vi "test_pathClassScalar.vi"(8 "error in (no error)":errorcluster) -> (0 "error out":errorcluster)   [LabVIEW 2020]
uses:
  test-TestableClass/Caraya-TestableClass.lvclass
  run-tests/Run Test (Scalar Path).vi
  Caraya.lvlib
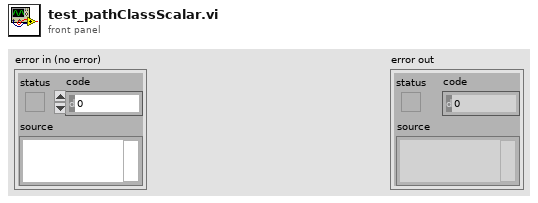
[diagram p1: front panel]
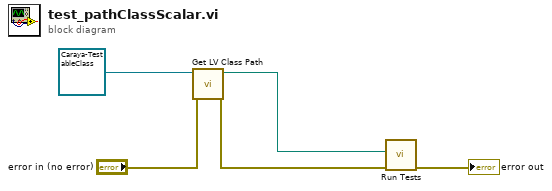
[diagram p0: block diagram]
diagram:
  n1 = call <vilib>:"Get LV Class Path.vi"("error in (no error)"="error in (no error)", "object"=refnum<class "Caraya-TestableClass.lvclass"> refnum ("Caraya-TestableClass.lvclass")) -> ("error out"=w2:errorcluster, "class path"=w4:path)  [unwired: 8 in]
  n2 = call-poly "Run Tests.vi"("error in"=w2, "Test Path"=w4) -> ("error out"=→"error out":errorcluster)  [unwired: 8 in, 1 out]
